vi "CAN Initialize.vi"(6 "Interrupt":u16, 7 "IOPort":u32, 8 "error in (no error)":errorcluster, 9 "HwType":u8, 10 "Btr0Btr1":u16, 11 "Channel":u16) -> (0 "error out":errorcluster, 3 "function return":u32)   [LabVIEW 2025, in "PCAN2023.lvlib"]
doc: "TPCANStatus __stdcall CAN_Initialize(\n TPCANHandle Channel, \n TPCANBaudrate Btr0Btr1, \n TPCANType HwType _DEF_ARG,\n DWORD IOPort _DEF_ARG, \n WORD Interrupt _DEF_ARG);"
uses:
  PCAN2023.lvlib
  x64/PCANBasic.dll
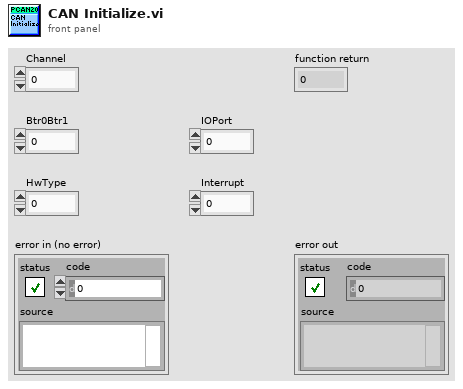
[diagram p1: front panel]
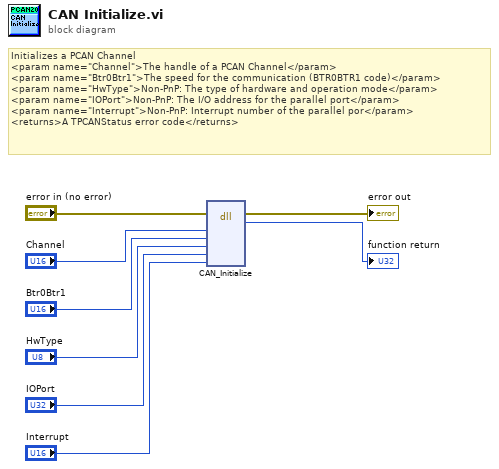
[diagram p0: block diagram]
diagram:
  # "Initializes a PCAN Channel \n<param name=\"Channel\">The handle of a PCAN Channel</param>\n<param name=\"Btr0Btr1\">The speed for the communication (BTR0BTR1 code)</param>\n<param name=\"HwType\">Non-PnP: The type of hardware and operation mode</param>\n<param name=\"IOPort\">Non-PnP: The I/O address for the parallel port</param>\n<param name=\"Interrupt\">Non-PnP: Interrupt number of the parallel por</param>\n<returns>A TPCANStatus error code</returns>"
  n1 = dll-call lib="C:/UTP/LabView/Communication Handle/PCAN2023/x64/PCANBasic.dll" fn="CAN_Initialize"(error in="error in (no error)", "Channel"="Channel", "Btr0Btr1"="Btr0Btr1", "HwType"="HwType", "IOPort"="IOPort", "Interrupt"="Interrupt") -> (error out=→"error out":errorcluster, "return type"=→"function return":u32)  [unwired: 7 in, 1 out]
